vi "UDP Time String to Date Time Rec.vi"() -> ()   [LabVIEW 2014]
uses:
  <vilib>/Utility/miscctls.llb/LVDateTimeRec.ctl
  myRIO/Controls/Switch Day.ctl
panel:
  out "output cluster":T1
  out "Day":string
  out "Second":i32
  out "Minute":i32
  out "Hour":i32
  in  "Time String":string
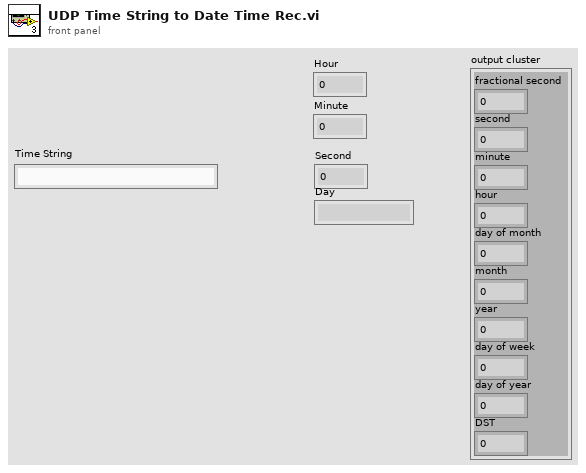
[diagram p1: front panel]
types:
  T1 = typedef "LVDateTimeRec.ctl" = cluster{"fractional second":dbl, "second":i32, "minute":i32, "hour":i32, "day of month":i32, "month":i32, "year":i32, "day of week":i32, "day of year":i32, "DST":i32}
  T2 = typedef "Switch Day.ctl" = enum16{"Eee", "Sun", "Mon", "Tue", "Wed", "Thu", "Fri", "Sat"}
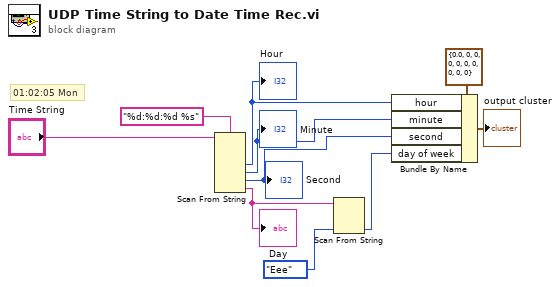
[diagram p0: block diagram]
diagram:
  # "01:02:05 Mon"
  n1 = Scan From String(format string="%d:%d:%d %s", input string="Time String") -> (output 1=w7:i32, output 2=w6:i32, output 3=w5:i32, output 4=w4:string)  [unwired: 6 in, 3 out]
  "Hour" <- w7
  "Minute" <- w6
  "Second" <- w5
  "Day" <- w4
  n2 = Scan From String(input string=w4, default 1=Switch_Day."Eee" ("Day")) -> (output 1=w2:T2)  [unwired: 3 in, 3 out]
  n3 = Bundle By Name(cluster=T1 {"fractional second"=0.0, "second"=0, "minute"=0, "hour"=0, "day of month"=0, "month"=0, "year"=0, "day of week"=0, "day of year"=0, "DST"=0} ("date time rec 2"), "hour"=w7, "minute"=w6, "second"=w5, "day of week"=w2) -> (→"output cluster":T1)
